vi "数值控件字号自适应.vi"(6 "留白（7）":i16=7, 7 "新旧尺寸信息":T1, 8 "错误输入（无错误）":errorcluster, 11 "数值控件-引用":refnum<vi>) -> (0 "错误输出":errorcluster, 3 "字号":u32)   [LabVIEW 2017]
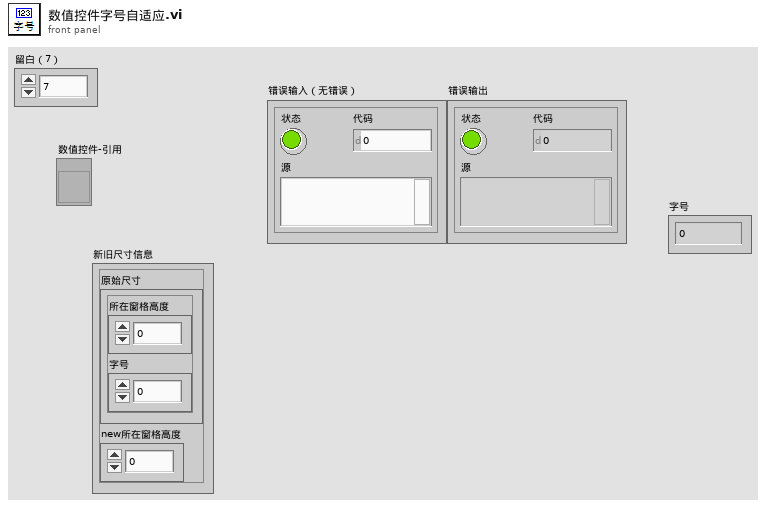
[diagram p1: front panel]
types:
  T1 = cluster{"原始尺寸":cluster{"所在窗格高度":u32, "字号":u32}, "new所在窗格高度":u32}
  T2 = typedef "LVRectTypeDef.ctl" = cluster{"Left":i16, "Top":i16, "Right":i16, "Bottom":i16}
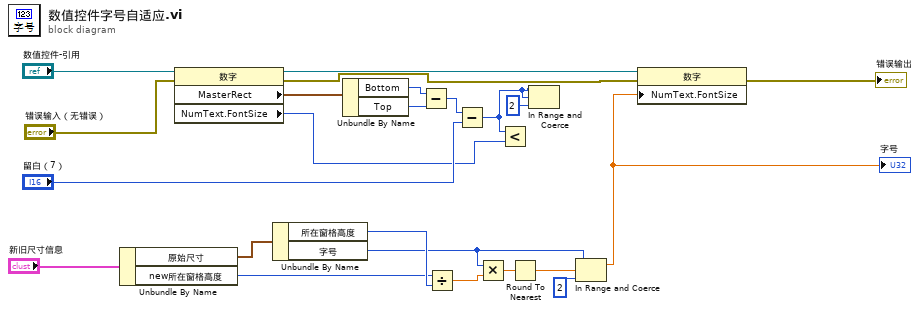
[diagram p0: block diagram]
diagram:
  n1 = Unbundle By Name("新旧尺寸信息") -> ("原始尺寸"=w6:cluster{"所在窗格高度":u32, "字号":u32}, "new所在窗格高度"=w7:u32)
  n2 = property class="数字"(reference="数值控件-引用", error in="错误输入（无错误）") -> (reference out=w14:refnum<vi>, error out=w21:errorcluster, "MasterRect"=w19:T2, "NumText.FontSize"=w13:u32)
  n3 = Unbundle By Name(w6) -> ("所在窗格高度"=w8:u32, "字号"=w3:u32)
  n4 = Unbundle By Name(w19) -> ("Bottom"=w17:i16, "Top"=w18:i16)
  n5 = Subtract(x=w17, y=w18) -> (x-y=w16:i16)
  n6 = Divide(x=w7, y=w8) -> (x/y=w9:dbl)
  n7 = Subtract(x=w16, y="留白（7）") -> (x-y=w11:i16)
  n8 = Multiply(x=w3, y=w9) -> (x*y=w10:dbl)
  n9 = Less?(x=w11, y=w13) -> ()  [unwired: 1 out]
  n10 = Round To Nearest(number=w10) -> (nearest integer value=w2:dbl)
  n11 = In Range and Coerce(upper limit=w11, x=w11, lower limit=i16 2 ("下限")) -> ()  [unwired: 2 out]
  n12 = In Range and Coerce(upper limit=w3, x=w2, lower limit=i16 2 ("下限")) -> (coerced(x)=w1:dbl)  [unwired: 1 out]
  "字号" <- w1
  n13 = property class="数字"(reference=w14, error in=w21, "NumText.FontSize"=w1) -> (error out=→"错误输出":errorcluster)  [unwired: 1 out]
